vi "print phase pgm.vi"(6 "max_val":i32=255, 7 "size_grid":dbl=0.02, 8 "gamma":dbl=1.0, 9 "n_grid":i32=256, 10 "Source Phase":path=path "C:/Users/Green Beret/Documents/Visual Studio 2012/Projects/LightPipes/LightPipes/lp12src/LabView/images/source_phase.pgm", 11 "Source Phase PGM":path=path "C:/Users/Green Beret/Documents/Visual Studio 2012/Projects/LightPipes/LightPipes/lp12src/LabView/images/source_phase.gpl") -> ()   [LabVIEW 2012, in "LightPipes.lvlib"]
uses:
  LightPipes.lvlib
panel:
  in  "lambda":dbl=1e-06
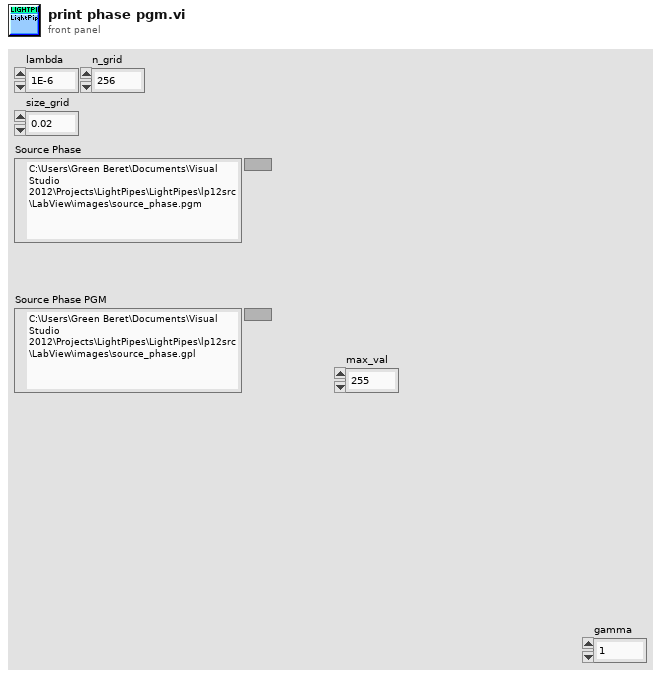
[diagram p1: front panel]
types:
  T1 = cluster{"n_grid":i32, "@dummy control@":i8, "@dummy control@":i8, "@dummy control@":i8, "@dummy control@":i8, "size":dbl, "lambda":dbl, "int1":i32, "int2":i32, "int3":i32, "@dummy control@":i8, "@dummy control@":i8, "@dummy control@":i8, "@dummy control@":i8, "double1":dbl, "double2":dbl, "double3":dbl, "real":u32, "imaginary":u32}
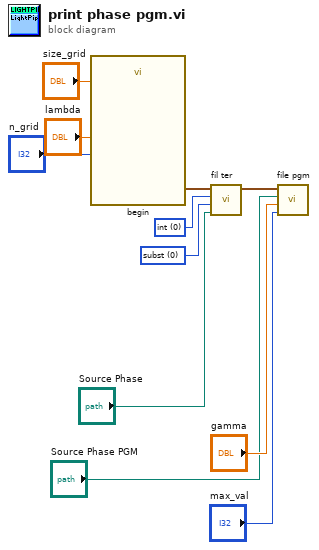
[diagram p0: block diagram]
diagram:
  w10 = i16 0 items=["subst", "mult"] ("multiplication/ substitution")
  w11 = i16 0 items=["int", "pha"] ("intensity / phase")
  n1 = call "begin.vi"("lambda"="lambda", "size_grid"="size_grid", "n_grid"="n_grid") -> ("field out"=w7:T1)  [unwired: 8 in]
  n2 = call "fil ter.vi"("Path"="Source Phase", "multiplication/ substitution"=w10, "intensity / phase"=w11, "field"=w7) -> ("field out"=w9:T1)  [unwired: 6 in, 1 out]
  n3 = call "file pgm.vi"("max_val"="max_val", "gamma"="gamma", "Path"="Source Phase PGM", "field"=w9) -> ()  [unwired: 6 in, 2 out]
